vi "BuildI2CTranscieveData.vi"(11 "Cluster":T1={"Port"=1, "I2CAdress"=1, "RX Length"=1, "Timeout"=1, "TX Data"=[]} {"TX Data" format="%04x"; "Timeout" format="%04d"; "RX Length" format="%04x"; "I2CAdress" format="%04x"; "Port" format="%04x"}) -> (2 "I2CDataAsString":string, 3 "I2CDataAsByteArray":u8[](array[numeric]))   [LabVIEW 2019]
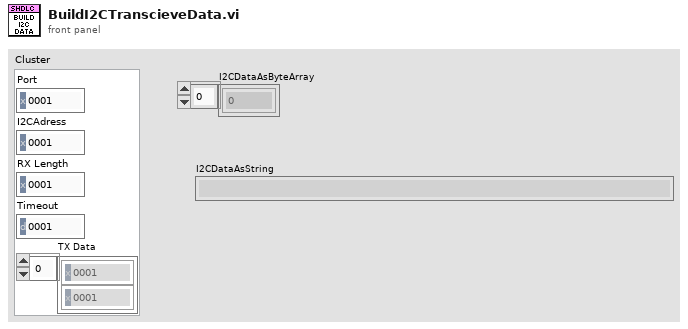
[diagram p1: front panel]
types:
  T1 = cluster{"Port":u8, "I2CAdress":u8, "RX Length":u32, "Timeout":u32, "TX Data":u8[]}
  T2 = enum16{"big-endian, network order", "native, host order", "little-endian"}
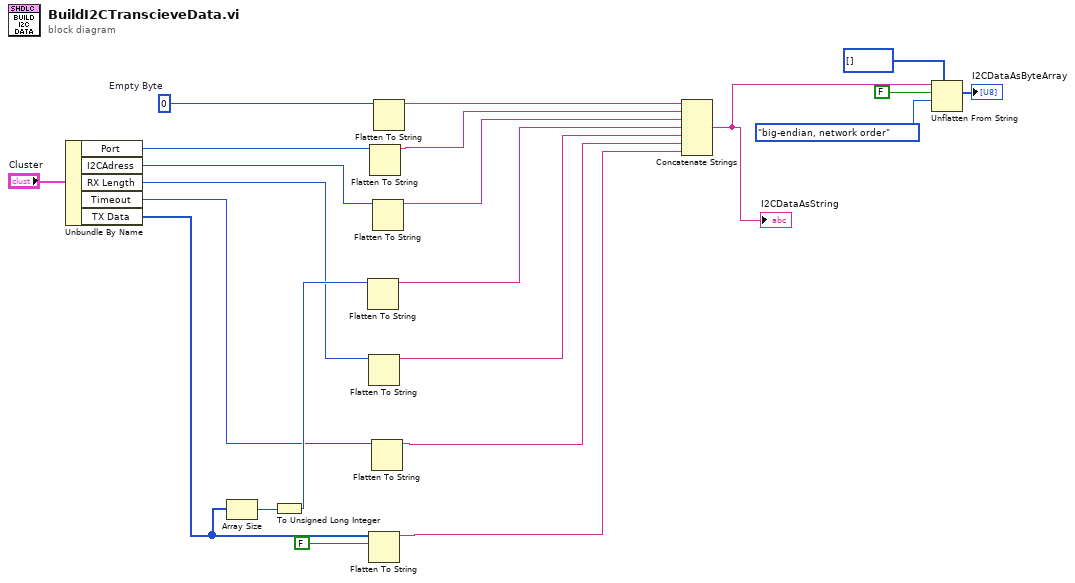
[diagram p0: block diagram]
diagram:
  w13 = u8 0  # Empty Byte
  n1 = Unbundle By Name("Cluster") -> ("Port"=w5:u8, "I2CAdress"=w4:u8, "RX Length"=w3:u32, "Timeout"=w2:u32, "TX Data"=w1:u8[])
  n2 = Array Size(array=w1) -> (size(s)=w16:i32)
  n3 = To Unsigned Long Integer(number=w16) -> (unsigned 32bit integer=w14:u32)
  n4 = Flatten To String(anything=w14) -> (data string=w20:string)  [unwired: 3 in, 2 out]
  n5 = Flatten To String(anything=w3) -> (data string=w19:string)  [unwired: 3 in, 2 out]
  n6 = Flatten To String(anything=w1, prepend array or string size? (T)=FALSE) -> (data string=w18:string)  [unwired: 2 in, 2 out]
  n7 = Flatten To String(anything=w5) -> (data string=w22:string)  [unwired: 3 in, 2 out]
  n8 = Flatten To String(anything=w2) -> (data string=w15:string)  [unwired: 3 in, 2 out]
  n9 = Flatten To String(anything=w4) -> (data string=w21:string)  [unwired: 3 in, 2 out]
  n10 = Flatten To String(anything=w13) -> (data string=w12:string)  [unwired: 3 in, 2 out]
  n11 = Concatenate Strings(w12, w22, w21, w20, w19, w15, w18) -> (w9:string)
  "I2CDataAsString" <- w9
  n12 = Unflatten From String(type=u8[] [] ("Array 2"), binary string=w9, data includes array or string size? (T)=FALSE, byte order (0:big-endian, network order)=T2."big-endian, network order") -> (value=→"I2CDataAsByteArray":u8[])  [unwired: 1 in, 2 out]
